vi "oa_Check Waveform (1 Channel).vi"(8 "error in (no error)":errorcluster, 11 "scaled signal [EU]":waveform(dbl)={"t0"=timestamp(0 s since 1904-01-01), "dt"=0.0, "Y"=[]}) -> (0 "error out":errorcluster, 1 "empty signal":bool, 3 "scaled signal [EU] out":waveform(dbl))   [LabVIEW 2017, in "SoundVib_Resampling.lvlib"]
uses:
  <vilib>/addons/Sound and Vibration/Order Analysis/Resample Order Tracking/SoundVib_Resampling.lvlib
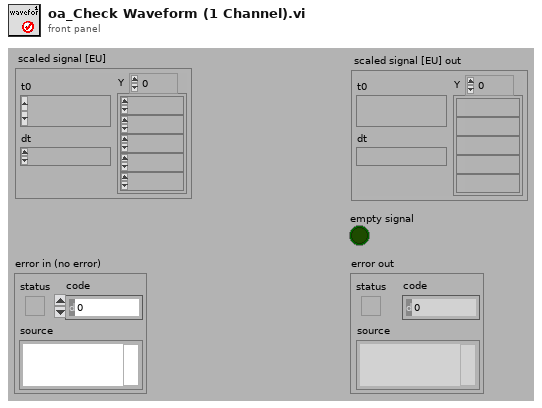
[diagram p1: front panel]
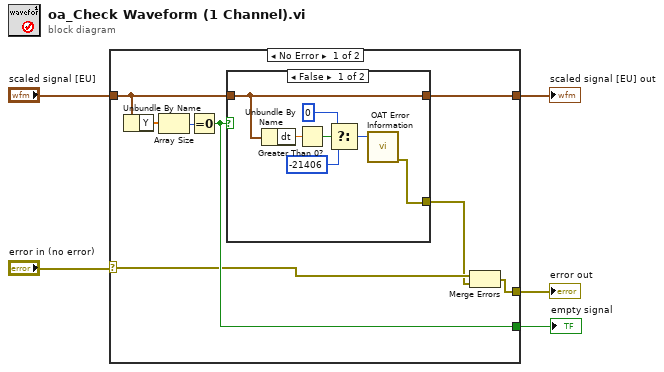
[diagram p0: block diagram]
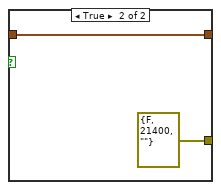
[diagram p2: hidden frame]
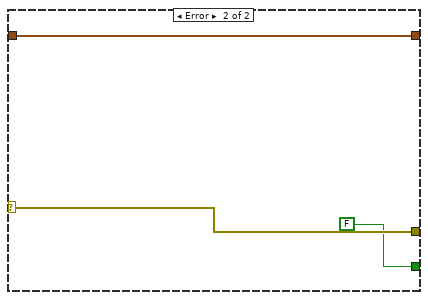
[diagram p3: hidden frame]
diagram:
  n1 = case shown="No Error" "error in (no error)" {
    selector: "error in (no error)" -> [w8 w25]
    tunnel: "scaled signal [EU]" -> [w11 w24]
    tunnel: [w6 w25] -> w3
    tunnel: [w10 w24] -> w2
    tunnel: [w9 FALSE] -> w1
    frame No Error {
      n2 = Unbundle By Name(w11) -> ("Y"=w13:dbl[])
      n3 = Array Size(array=w13) -> (size(s)=w12:i32)
      n4 = Equal To 0?(x=w12) -> (x = 0?=w9:bool)
      n5 = case shown="False" w9 {
        tunnel: w11 -> [w14 w21]
        tunnel: [w15 errorcluster {"status"=FALSE, "code"=21400, "source"=""} ("error in (no error)")] -> w7
        tunnel: [w14 w21] -> w10
        frame False {
          n6 = Unbundle By Name(w14) -> ("dt"=w20:dbl)
          n7 = Greater Than 0?(x=w20) -> (x > 0?=w19:bool)
          n8 = Select(t=0 ("code"), s=w19, f=-21406 ("code")) -> (s? t:f=w16:i32)
          n9 = call <vilib>:"OAT Error Information.vi"("error code"=w16) -> ("error out"=w15:errorcluster)  [unwired: 6 in]
        }
        frame True {
        }
      }
      n10 = Merge Errors(w8, w7) -> (w6:errorcluster)
    }
    frame Error {
    }
  }
  "error out" <- w3
  "scaled signal [EU] out" <- w2
  "empty signal" <- w1
